vi "Perform Step.vi"(8 "error in (no error)":errorcluster, 11 "String Assertion in":refnum<class "String Assertion.lvclass">) -> (0 "error out":errorcluster, 2 "Result":T1, 3 "String Assertion out":refnum<class "String Assertion.lvclass">)   [LabVIEW 2020, in "MacroAssert.lvlib" / "String Assertion.lvclass"]
doc: "Performs all actions required for <B>Step in</B>."
uses:
  String Assertion.lvclass
  String Assertion.lvclass/String Assertion.ctl
  CTLs/Report Data.ctl
  MacroAssert.lvlib
  SubVIs/Win Util/Win Util.lvlib
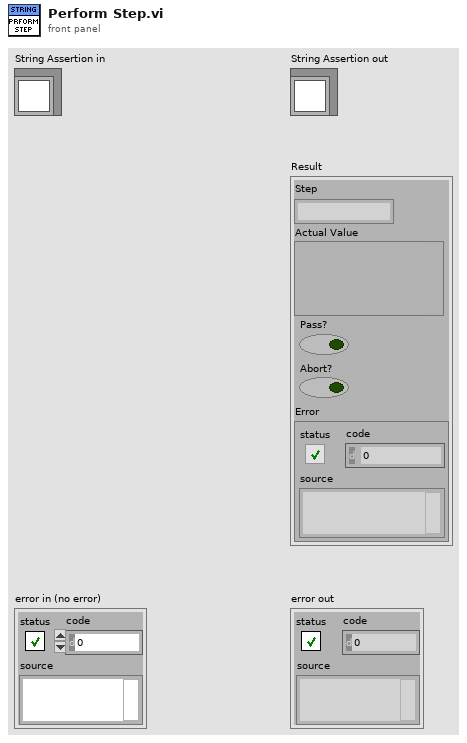
[diagram p1: front panel]
types:
  T1 = typedef "MacroAssert.lvlib/Report Data.ctl" = cluster{"Step":string, "Actual Value":variant, "Pass?":bool, "Abort?":bool, "Error":errorcluster}
  T2 = typedef "MacroAssert.lvlib/String Assertion.lvclass/String Comparator.ctl" = enum16{"Contains", "Equals", "Starts with", "Ends with", "Does not contain", "Does not equal"}
  T3 = typedef "MacroAssert.lvlib/String Assertion.lvclass/String Assertion Type.ctl" = enum16{"String Ctl Value", "Ctl Caption Property", "Ctl Tip Strip Property", "Frontmost VI Name", "Frontmost Window Name"}
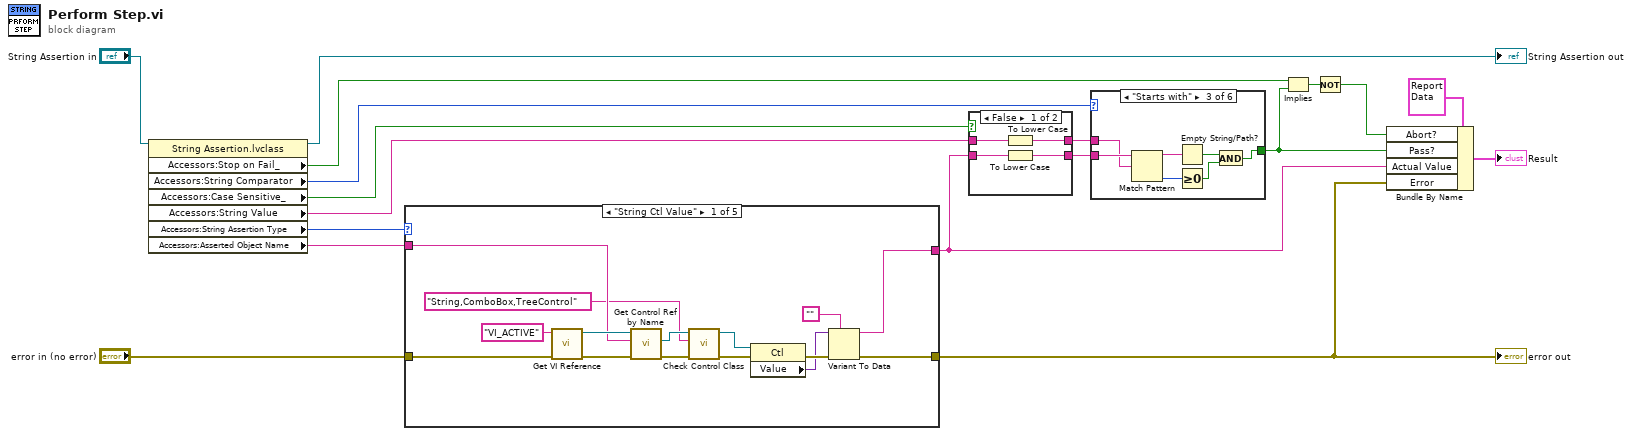
[diagram p0: block diagram]
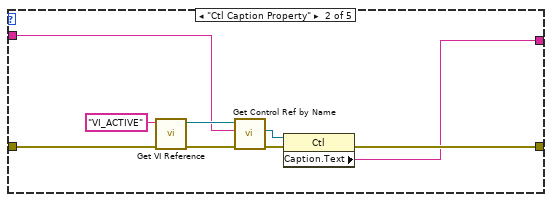
[diagram p3: hidden frame]
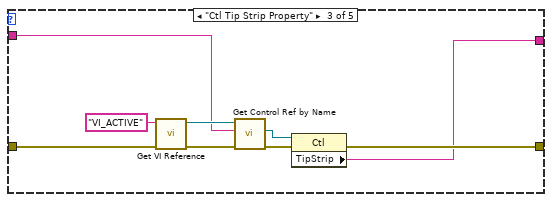
[diagram p4: hidden frame]
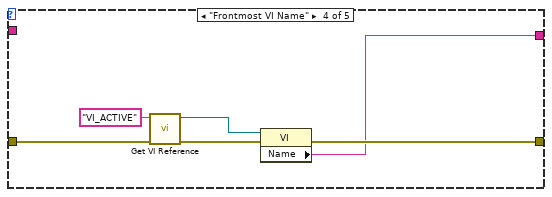
[diagram p5: hidden frame]
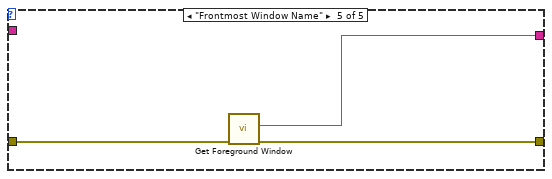
[diagram p6: hidden frame]
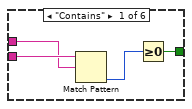
[diagram p7: hidden frame]
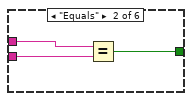
[diagram p8: hidden frame]
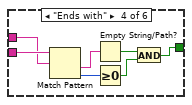
[diagram p9: hidden frame]
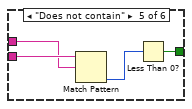
[diagram p10: hidden frame]
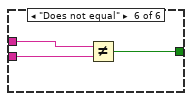
[diagram p11: hidden frame]
diagram:
  n1 = property class="String Assertion.lvclass"(reference="String Assertion in") -> (reference out=→"String Assertion out":refnum<class "String Assertion.lvclass">, "Accessors:Stop on Fail_"=w9:bool, "Accessors:String Comparator"=w12:T2, "Accessors:Case Sensitive_"=w5:bool, "Accessors:String Value"=w4:string, "Accessors:String Assertion Type"=w17:T3, "Accessors:Asserted Object Name"=w18:string)  [unwired: 1 in, 1 out]
  n2 = case shown="\"String Ctl Value\"" w17 {
    tunnel: "error in (no error)" -> [w32 w40 w49 w57 w60]
    tunnel: [w30 w39 w48 w55 w59] -> w6
    tunnel: w18 -> [w28 w36 w45 _ _]
    tunnel: [w25 w35 w44 w53 w58] -> w1
    frame "String Ctl Value" {
      n3 = call "Get VI Reference.vi"("error in (no error)"=w32, "VI Name"="VI_ACTIVE") -> ("error out"=w33:errorcluster, "VI Ref"=w29:refnum<vi>)  [unwired: 8 in]
      n4 = call "Get Control Ref by Name.vi"("error in (no error)"=w33, "Name"=w28, "VI Ref"=w29) -> ("error out"=w24:errorcluster, "Ctl Ref"=w22:refnum<vi>)  [unwired: 6 in, 1 out]
      n5 = call "Check Control Class.vi"("error in (no error)"=w24, "Supported Classes"="String,ComboBox,TreeControl", "Ctl Ref"=w22) -> ("error out"=w23:errorcluster, "Ctl Ref out"=w20:refnum<vi>)  [unwired: 7 in]
      n6 = property class="Ctl"(reference=w20, error in=w23) -> (error out=w31:errorcluster, "Value"=w26:variant)  [unwired: 1 out]
      n7 = Variant To Data(error in=w31, type="", Variant=w26) -> (data=w25:string, error out=w30:errorcluster)
    }
    frame "Ctl Caption Property" {
      n8 = call "Get VI Reference.vi"("error in (no error)"=w40, "VI Name"="VI_ACTIVE") -> ("error out"=w42:errorcluster, "VI Ref"=w38:refnum<vi>)  [unwired: 8 in]
      n9 = call "Get Control Ref by Name.vi"("error in (no error)"=w42, "Name"=w36, "VI Ref"=w38) -> ("error out"=w41:errorcluster, "Ctl Ref"=w37:refnum<vi>)  [unwired: 6 in, 1 out]
      n10 = property class="Ctl"(reference=w37, error in=w41) -> (error out=w39:errorcluster, "Caption.Text"=w35:string)  [unwired: 1 out]
    }
    frame "Ctl Tip Strip Property" {
      n11 = call "Get VI Reference.vi"("error in (no error)"=w49, "VI Name"="VI_ACTIVE") -> ("error out"=w51:errorcluster, "VI Ref"=w47:refnum<vi>)  [unwired: 8 in]
      n12 = call "Get Control Ref by Name.vi"("error in (no error)"=w51, "Name"=w45, "VI Ref"=w47) -> ("error out"=w50:errorcluster, "Ctl Ref"=w46:refnum<vi>)  [unwired: 6 in, 1 out]
      n13 = property class="Ctl"(reference=w46, error in=w50) -> (error out=w48:errorcluster, "TipStrip"=w44:string)  [unwired: 1 out]
    }
    frame "Frontmost VI Name" {
      n14 = call "Get VI Reference.vi"("error in (no error)"=w57, "VI Name"="VI_ACTIVE") -> ("error out"=w56:errorcluster, "VI Ref"=w54:refnum<vi>)  [unwired: 8 in]
      n15 = property class="VI"(reference=w54, error in=w56) -> (error out=w55:errorcluster, "Name"=w53:string)  [unwired: 1 out]
    }
    frame "Frontmost Window Name" {
      n16 = call "Get Foreground Window.vi"("error in (no error)"=w60) -> ("error out"=w59:errorcluster, "window name"=w58:string)  [unwired: 8 in, 1 out]
    }
  }
  "error out" <- w6
  n17 = case shown="False" w5 {
    tunnel: w4 -> [w64 w66]
    tunnel: [w62 w66] -> w3
    tunnel: [w61 w65] -> w2
    tunnel: w1 -> [w63 w65]
    frame False {
      n18 = To Lower Case(string=w64) -> (all lower case string=w62:string)
      n19 = To Lower Case(string=w63) -> (all lower case string=w61:string)
    }
    frame True {
    }
  }
  n20 = case shown="\"Starts with\"" w12 {
    tunnel: w3 -> [w69 w73 w79 w86 w90 w94]
    tunnel: [w68 w72 w76 w84 w89 w93] -> w8
    tunnel: w2 -> [w70 w71 w80 w87 w91 w92]
    frame "Contains" {
      n21 = Match Pattern(string=w70, regular expression=w69) -> (offset past match=w67:i32)  [unwired: 1 in, 3 out]
      n22 = Greater Or Equal To 0?(x=w67) -> (x >= 0?=w68:bool)
    }
    frame "Equals" {
      n23 = Equal?(x=w73, y=w71) -> (x = y?=w72:bool)
    }
    frame "Starts with" {
      n24 = Match Pattern(string=w80, regular expression=w79) -> (before substring=w78:string, offset past match=w77:i32)  [unwired: 1 in, 2 out]
      n25 = Empty String/Path?(string/path=w78) -> (empty?=w75:bool)
      n26 = Greater Or Equal To 0?(x=w77) -> (x >= 0?=w74:bool)
      n27 = And(x=w75, y=w74) -> (x .and. y?=w76:bool)
    }
    frame "Ends with" {
      n28 = Match Pattern(string=w87, regular expression=w86) -> (after substring=w81:string, offset past match=w85:i32)  [unwired: 1 in, 2 out]
      n29 = Empty String/Path?(string/path=w81) -> (empty?=w83:bool)
      n30 = Greater Or Equal To 0?(x=w85) -> (x >= 0?=w82:bool)
      n31 = And(x=w83, y=w82) -> (x .and. y?=w84:bool)
    }
    frame "Does not contain" {
      n32 = Match Pattern(string=w91, regular expression=w90) -> (offset past match=w88:i32)  [unwired: 1 in, 3 out]
      n33 = Less Than 0?(x=w88) -> (x < 0?=w89:bool)
    }
    frame "Does not equal" {
      n34 = Not Equal?(x=w94, y=w92) -> (x != y?=w93:bool)
    }
  }
  n35 = Implies(1:w8, 2:w9) -> (0:w10:bool)
  n36 = Not(x=w10) -> (.not. x?=w7:bool)
  n37 = Bundle By Name(cluster=T1 {"Step"="", "Actual Value"=variant, "Pass?"=FALSE, "Abort?"=FALSE, "Error"={"status"=FALSE, "code"=0, "source"=""}} ("Report Data"), "Abort?"=w7, "Pass?"=w8, "Actual Value"=w1, "Error"=w6) -> (→"Result":T1)
